vi "Initialize.vi"(8 "error in (no error)":errorcluster, 10 "Temp Conotroller Config":T1={"COM Port"="COM14", "Type"=enum."Disabled"}, 11 "Temperature Controller in":refnum<class "Temperature Controller.lvclass">) -> (0 "error out":errorcluster, 3 "Temperature Controller out":refnum<class "Temperature Controller.lvclass">)   [LabVIEW 2023, in "Temperature Controller.lvlib" / "Temperature Controller.lvclass"]
uses:
  Temperature Controller.lvclass
  Resources/Type Defs/Temp Controller Configuration.ctl
  Temperature Controller.lvclass/Temperature Controller.ctl
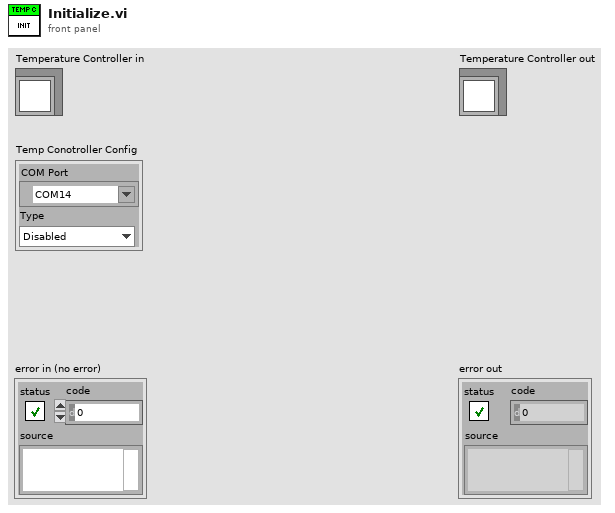
[diagram p1: front panel]
types:
  T1 = typedef "Temp Controller Configuration.ctl" = cluster{"COM Port":refnum<visa-resource-name>, "Type":enum16{"Disabled", "TC-720"}}
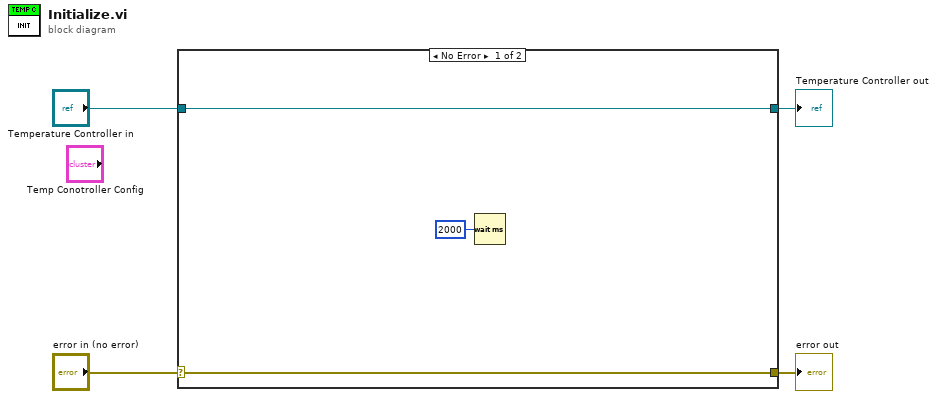
[diagram p0: block diagram]
diagram:
  n1 = case shown="No Error" "error in (no error)" {
    selector: "error in (no error)" -> [w6 w9]
    tunnel: [w6 w9] -> w3
    tunnel: [w7 w8] -> w1
    tunnel: "Temperature Controller in" -> [w7 w8]
    frame No Error {
      n2 = Wait (ms)(milliseconds to wait=u32 2000) -> ()  [unwired: 1 out]
    }
    frame Error {
    }
  }
  "error out" <- w3
  "Temperature Controller out" <- w1
